vi "Trigger conf.vi"(7 "Source (auto)":T1, 8 "error in (no error)":errorcluster, 9 "Interval (100ms)":u32=100 min=8 max=2000 step=1, 11 "Reference in":T2={"Device"="GPIB0::4::INSTR", "Function"="", "delay"=20}) -> (0 "error out":errorcluster, 3 "Reference out":T2={"Device"="GPIB0::4::INSTR", "Function"="", "delay"=20}, 4 "question out":string)   [LabVIEW 2021, in "Rigol DM3052.lvlib"]
uses:
  Rigol DM3052.lvlib
  Reference.ctl
  Trig sources.ctl
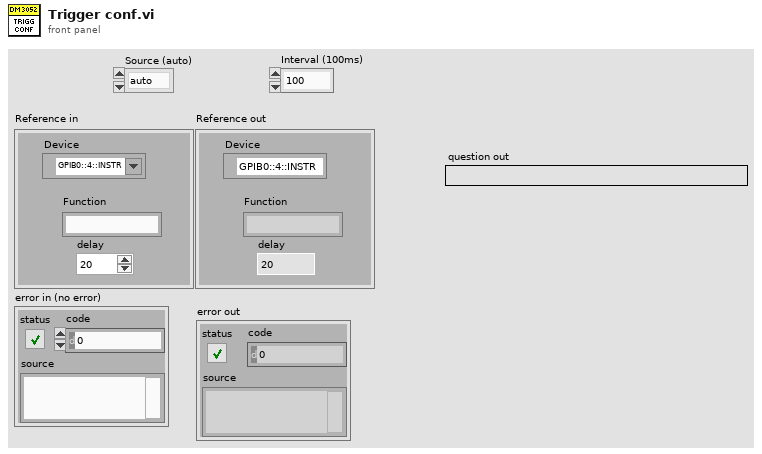
[diagram p1: front panel]
types:
  T1 = typedef "Rigol DM3052.lvlib/Trig sources.ctl" = enum16{"auto", "single", "ext"}
  T2 = typedef "Rigol DM3052.lvlib/Reference.ctl" = cluster{"Device":refnum<visa-resource-name>, "Function":string, "delay":u32}
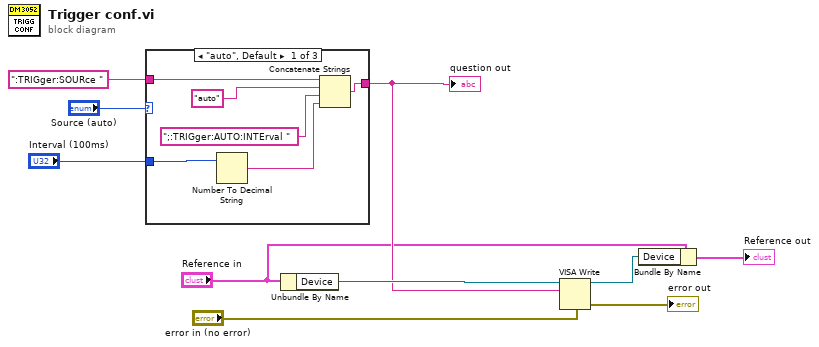
[diagram p0: block diagram]
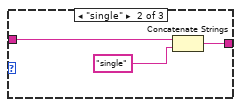
[diagram p2: hidden frame]
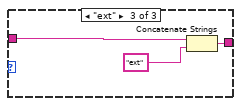
[diagram p3: hidden frame]
diagram:
  n1 = case shown="\"auto\", Default" "Source (auto)" {
    tunnel: ":TRIGger:SOURce " -> [w15 w18 w21]
    tunnel: [w14 w17 w20] -> w4
    tunnel: "Interval (100ms)" -> [w12 _ _]
    frame "auto", Default {
      n2 = Number To Decimal String(number=w12) -> (decimal integer string=w11:string)  [unwired: 1 in]
      n3 = Concatenate Strings(w15, "auto", ";:TRIGger:AUTO:INTErval ", w11) -> (w14:string)
    }
    frame "single" {
      n4 = Concatenate Strings(w18, "single") -> (w17:string)
    }
    frame "ext" {
      n5 = Concatenate Strings(w21, "ext") -> (w20:string)
    }
  }
  "question out" <- w4
  n6 = Unbundle By Name("Reference in") -> ("Device"=w9:refnum<visa-resource-name>)
  n7 = VISA Write(VISA resource name=w9, write buffer=w4, error in (no error)="error in (no error)") -> (VISA resource name out=w2:refnum<visa-resource-name>, error out=→"error out":errorcluster)  [unwired: 1 out]
  n8 = Bundle By Name(cluster="Reference in", "Device"=w2) -> (→"Reference out":T2)
